vi "Dynamixel.vi"(0 "ID":u8, 1 "Instruction":u8, 3 "Array in":u8[](array[numeric])) -> (7 "Array out":u8[](array[numeric]))   [LabVIEW 2019]
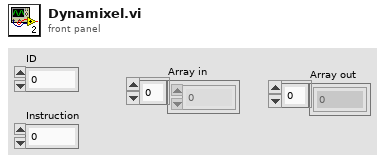
[diagram p1: front panel]
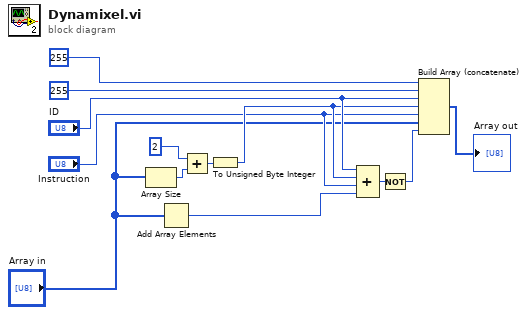
[diagram p0: block diagram]
diagram:
  n1 = Array Size(array="Array in") -> (size(s)=w10:i32)
  n2 = Add Array Elements(numeric array="Array in") -> (sum=w1:u8)
  n3 = Add(x=2, y=w10) -> (x+y=w8:i32)
  n4 = To Unsigned Byte Integer(number=w8) -> (unsigned 8bit integer=w6:u8)
  n5 = Compound Arithmetic op=ADD("ID", w6, "Instruction", w1) -> (w4:u8)
  n6 = Not(x=w4) -> (.not. x?=w2:u8)
  n7 = Build Array (concatenate)(u8 255, u8 255, "ID", w6, "Instruction", "Array in", w2) -> (→"Array out":u8[])
